vi "Calculate_Vector_length_brasse.vi"(8 "Vector 2 z":dbl, 9 "Vector 2 y":dbl, 10 "Vector 1 z":dbl, 11 "Vector 1 y":dbl) -> (3 "Length":dbl)   [LabVIEW 2009]
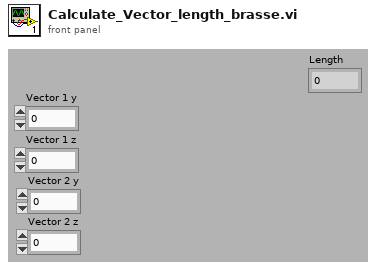
[diagram p1: front panel]
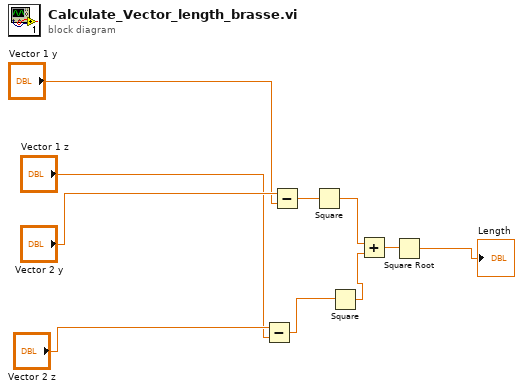
[diagram p0: block diagram]
diagram:
  n1 = Subtract(x="Vector 2 z", y="Vector 1 z") -> (x-y=w5:dbl)
  n2 = Subtract(x="Vector 2 y", y="Vector 1 y") -> (x-y=w6:dbl)
  n3 = Square(x=w6) -> (x^2=w3:dbl)
  n4 = Square(x=w5) -> (x^2=w4:dbl)
  n5 = Add(x=w3, y=w4) -> (x+y=w2:dbl)
  n6 = Square Root(x=w2) -> (sqrt(x)=→"Length":dbl)
